vi "Retrieve Config.vi"(8 "error in":errorcluster, 11 "Artifactory":refnum<class "Artifactory.lvclass">) -> (0 "error out":errorcluster, 2 "Config":T1, 3 "Artifactory out":refnum<class "Artifactory.lvclass">, 5 "found":bool)   [LabVIEW 2021, in "Artifactory.lvclass"]
uses:
  Artifactory.lvclass
  Config -- cluster.ctl
  39216332-d583-4564-a6e2-ab2ce037b1bf.vi
  <vilib>/Utility/error.llb/Error Cluster From Error Code.vi
  <vilib>/JDP Science/JSONtext/JSON text to Variant.vi
  <vilib>/ErrorRing/Error Ring.xnode
  <vilib>/JDP Science/JSONtext/LVClass Serializer/JSONtext LVClass Serializer.lvclass
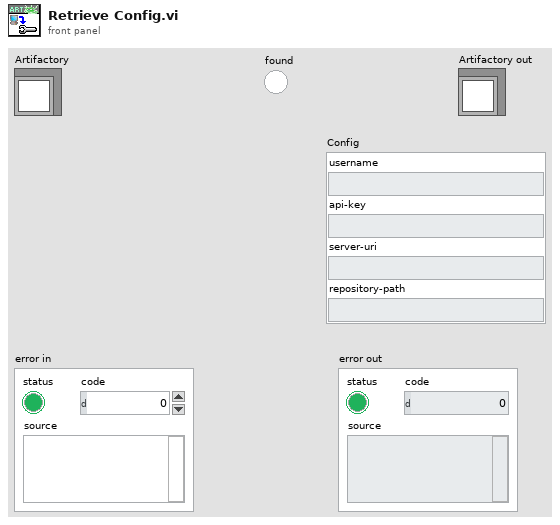
[diagram p1: front panel]
types:
  T1 = typedef "Artifactory.lvclass/Config -- cluster.ctl" = cluster{"username":string, "api-key":string, "server-uri":string, "repository-path":string}
  T2 = enum16{"open", "replace", "create", "open or create", "replace or create", "replace or create with confirmation"}
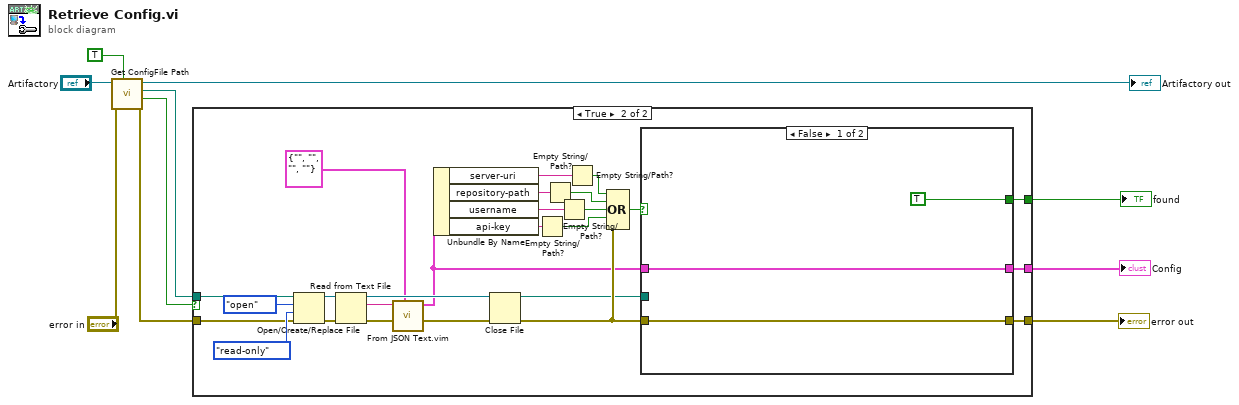
[diagram p0: block diagram]
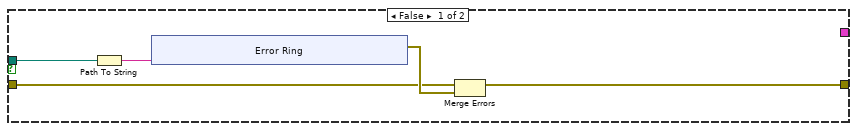
[diagram p2: hidden frame]
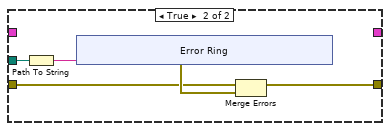
[diagram p3: hidden frame]
diagram:
  n1 = call-dynamic "Get ConfigFile Path.vi"("create folder? (T)"=TRUE, "error in (no error)"="error in", "Artifactory in"="Artifactory") -> ("error out"=w8:errorcluster, "found"=w7:bool, "Config File"=w6:path, "Artifactory out"=→"Artifactory out":refnum<class "Artifactory.lvclass">)  [unwired: 5 in]
  n2 = case shown="True" w7 {
    tunnel: [w14 w38] -> w2
    tunnel: [_ w33] -> w1
    tunnel: w8 -> [w13 w40]
    tunnel: w6 -> [w12 w39]
    tunnel: [_ w32] -> w4
    frame False {
      n3 = Path To String(path=w12) -> (string=w11:string)
      n4 = xnode "Error Ring"("parameter 0"=w11) -> ("error out"=w15:errorcluster)
      n5 = Merge Errors(w13, w15) -> (w14:errorcluster)
    }
    frame True {
      n6 = Open/Create/Replace File(file path (use dialog)=w39, error in=w40, operation (0:open)=T2."open", access (0:read/write)=enum16{"read/write", "read-only", "write-only"}."read-only") -> (refnum out=w48:refnum<file>, error out=w46:errorcluster)  [unwired: 2 in, 1 out]
      n7 = Read from Text File(file (use dialog)=w48, error in=w46) -> (refnum out=w45:refnum<file>, text=w43:string, error out=w42:errorcluster)  [unwired: 2 in, 1 out]
      n8 = call "From JSON Text.vim"("Data Type and Default Value"=T1 {"username"="", "api-key"="", "server-uri"="", "repository-path"=""} ("Config"), "error in (no error)"=w42, "JSON"=w43) -> ("error out"=w41:errorcluster, "Data out"=w30:T1)  [unwired: 7 in]
      n9 = Unbundle By Name(w30) -> ("server-uri"=w25:string, "repository-path"=w26:string, "username"=w34:string, "api-key"=w35:string)
      n10 = Close File(refnum=w45, error in=w41) -> (path=w28:path, error out=w31:errorcluster)
      n11 = Empty String/Path?(string/path=w35) -> (empty?=w29:bool)
      n12 = Empty String/Path?(string/path=w26) -> (empty?=w24:bool)
      n13 = Empty String/Path?(string/path=w34) -> (empty?=w37:bool)
      n14 = Empty String/Path?(string/path=w25) -> (empty?=w23:bool)
      n15 = Compound Arithmetic op=OR(w23, w24, w37, w29, w31) -> (w36:bool)
      n16 = case shown="False" w36 {
        tunnel: w31 -> [w51 w55]
        tunnel: [w51 w54] -> w38
        tunnel: [w49 _] -> w33
        tunnel: [TRUE _] -> w32
        tunnel: w30 -> [w49 _]
        tunnel: w28 -> [_ w53]
        frame False {
        }
        frame True {
          n17 = Path To String(path=w53) -> (string=w52:string)
          n18 = xnode "Error Ring"("parameter 0"=w52) -> ("error out"=w56:errorcluster)
          n19 = Merge Errors(w55, w56) -> (w54:errorcluster)
        }
      }
    }
  }
  "error out" <- w2
  "Config" <- w1
  "found" <- w4
